vi "Read LoginResponse.vi"(8 "error in (no error)":errorcluster, 11 "UserInfo in":refnum<class "UserInfo.lvclass">) -> (0 "error out":errorcluster, 2 "LoginResponse":cluster{"UserInfo":T1, "PassWordExists？":bool}, 3 "UserInfo out":refnum<class "UserInfo.lvclass">)   [LabVIEW 2019, in "UserManagement.lvlib" / "UserInfo.lvclass"]
uses:
  UserInfo.lvclass
  UserInfo.ctl
  Permission.ctl
  UserInfo.lvclass/UserInfo.ctl
  UserManagement.lvclass
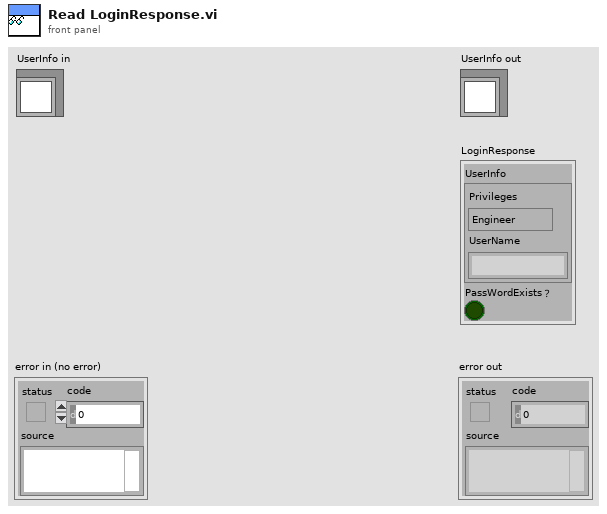
[diagram p1: front panel]
types:
  T1 = typedef "UserManagement.lvlib/UserManagement.lvclass/UserInfo.ctl" = cluster{"Privileges":T2, "UserName":string}
  T2 = typedef "UserManagement.lvlib/UserManagement.lvclass/Permission.ctl" = enum16{"Engineer", "Technical", "Operator"}
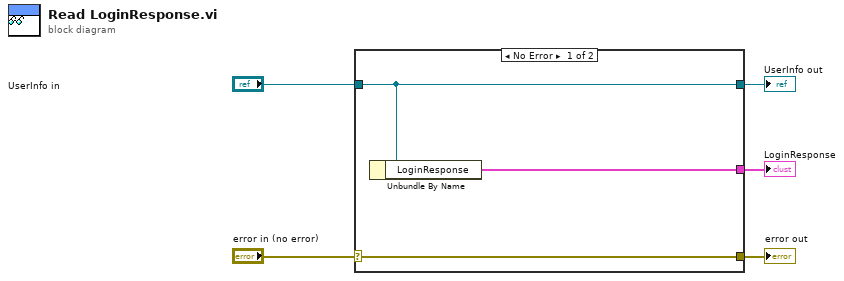
[diagram p0: block diagram]
diagram:
  n1 = case shown="No Error" "error in (no error)" {
    selector: "error in (no error)" -> [w8 w9]
    tunnel: [w8 w9] -> w4
    tunnel: [w7 w10] -> w2
    tunnel: "UserInfo in" -> [w7 w10]
    tunnel: [w6 _] -> w1
    frame No Error {
      n2 = Unbundle By Name(w7) -> ("LoginResponse"=w6:cluster{"UserInfo":T1, "PassWordExists？":bool})
    }
    frame Error {
    }
  }
  "error out" <- w4
  "UserInfo out" <- w2
  "LoginResponse" <- w1
